vi "Test SG.vi"() -> ()   [LabVIEW 2020, in "Signal Generator.lvclass"]
uses:
  Signal Generator.lvclass
  PSG-MXG/PSG-MXG.lvclass
  C:/Sandbox/Git_Sandbox/WiSpry Test Framework source code (LV20)/WiSpry Test Framework/Instruments/Instrument.lvclass
  Instrument.lvclass/Instrument.ctl
  Instrument.lvclass
panel:
  in  "VISA resource name":refnum<visa-resource-name>
  in  "Reset":bool
  in  "Frequency [Hz]":dbl=1000000000.0
  in  "Output Power [dBm]":dbl=-20.0
  in  "Output Enable (F)":bool
  out "Instrument out":refnum<class "PSG-MXG.lvclass">
  out "error out":errorcluster
  in  "Go Local (\"@LOC\")":bool=TRUE
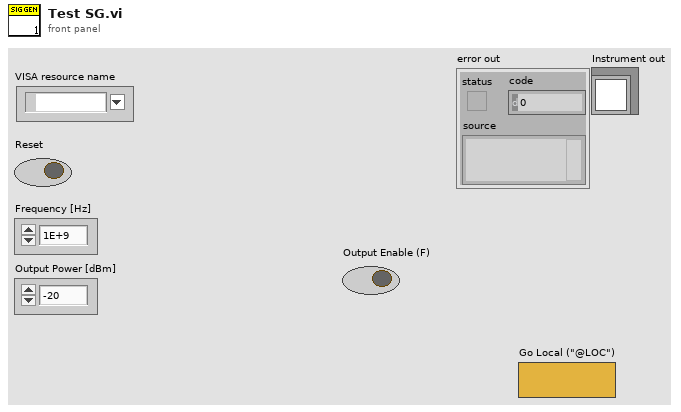
[diagram p1: front panel]
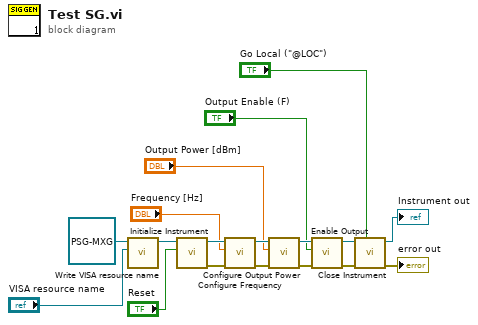
[diagram p0: block diagram]
diagram:
  n1 = call "Write VISA resource name.vi"("VISA resource name"="VISA resource name", "Instrument in"=refnum<class "PSG-MXG.lvclass"> refnum ("PSG-MXG.lvclass")) -> ("Instrument out"=w17:refnum<class "PSG-MXG.lvclass">)  [unwired: 9 in]
  n2 = call-dynamic "Initialize Instrument.vi"("Reset"="Reset", "PSG-MXG in"=w17) -> ("error out"=w15:errorcluster, "PSG-MXG out"=w16:refnum<class "PSG-MXG.lvclass">)  [unwired: 8 in]
  n3 = call-dynamic "Configure Frequency.vi"("error in (no error)"=w15, "Frequency [Hz]"="Frequency [Hz]", "PSG-MXG in"=w16) -> ("error out"=w13:errorcluster, "PSG-MXG out"=w14:refnum<class "PSG-MXG.lvclass">)  [unwired: 7 in]
  n4 = call-dynamic "Configure Output Power.vi"("error in (no error)"=w13, "Output Power [dBm]"="Output Power [dBm]", "PSG-MXG in"=w14) -> ("error out"=w11:errorcluster, "PSG-MXG out"=w12:refnum<class "PSG-MXG.lvclass">)  [unwired: 7 in]
  n5 = call-dynamic "Enable Output.vi"("error in (no error)"=w11, "Output Enable (F)"="Output Enable (F)", "PSG-MXG in"=w12) -> ("error out"=w9:errorcluster, "PSG-MXG out"=w10:refnum<class "PSG-MXG.lvclass">)  [unwired: 7 in]
  n6 = call-dynamic "Close Instrument.vi"("Go Local (\"@LOC\")"="Go Local (\"@LOC\")", "error in (no error)"=w9, "Instrument in"=w10) -> ("error out"=→"error out":errorcluster, "Instrument out"=→"Instrument out":refnum<class "PSG-MXG.lvclass">)  [unwired: 7 in]
